vi "Attack Action.vi"(11 "Direction":T1) -> (3 "Run Result":T2)   [LabVIEW 2020, in "SquareBattle.lvlib"]
uses:
  SquareBattle.lvlib
  Run Result.ctl
  Square/Square.lvclass
  Action.ctl
  Direction.ctl
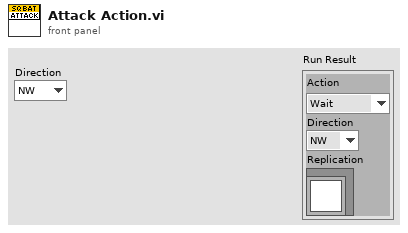
[diagram p1: front panel]
types:
  T1 = typedef "SquareBattle.lvlib/Direction.ctl" = enum16{"NW", "N", "NE", "E", "SE", "S", "SW", "W"}
  T2 = typedef "SquareBattle.lvlib/Run Result.ctl" = cluster{"Action":T3, "Direction":T1, "Replication":refnum<class "Square.lvclass">}
  T3 = typedef "SquareBattle.lvlib/Action.ctl" = enum16{"Wait", "Move", "Attack", "Replicate"}
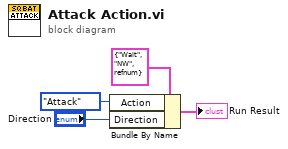
[diagram p0: block diagram]
diagram:
  n1 = Bundle By Name(cluster=T2 {"Action"=enum."Wait", "Direction"=enum."NW", "Replication"=refnum} ("Run Result"), "Action"=Action."Attack", "Direction"="Direction") -> (→"Run Result":T2)
